vi "SM-SG Main.vi"() -> ()   [LabVIEW 2017]
doc: "Use this template to build a simple state machine design pattern. Each state executes code and determines which state to transition to."
uses:
  controls/SM-SG State.ctl
  controls/SM-SG Data.ctl
  <vilib>/Waveform/WDTOps.llb/WDT Append Waveforms DBL.vi
  <vilib>/measure/NI_MABase.lvlib
panel:
  in  "Parâmetros Onda Trapezoidal":T1
  in  "Parâmetros de Geração":T2
  in  "Configurações da Onda":T3
  out "Sinal":waveform(dbl)(graph)={"t0"=timestamp(0 s since 1904-01-01), "dt"=0.0002, "Y"=[]}
  out "Onda":dbl[](graph)
  in  "Abrir":bool
  in  "Salvar":bool
  in  "Limpa":bool
  in  "Adicionar":bool
  in  "Stop Button":bool
  # "Gerador de Sinais"
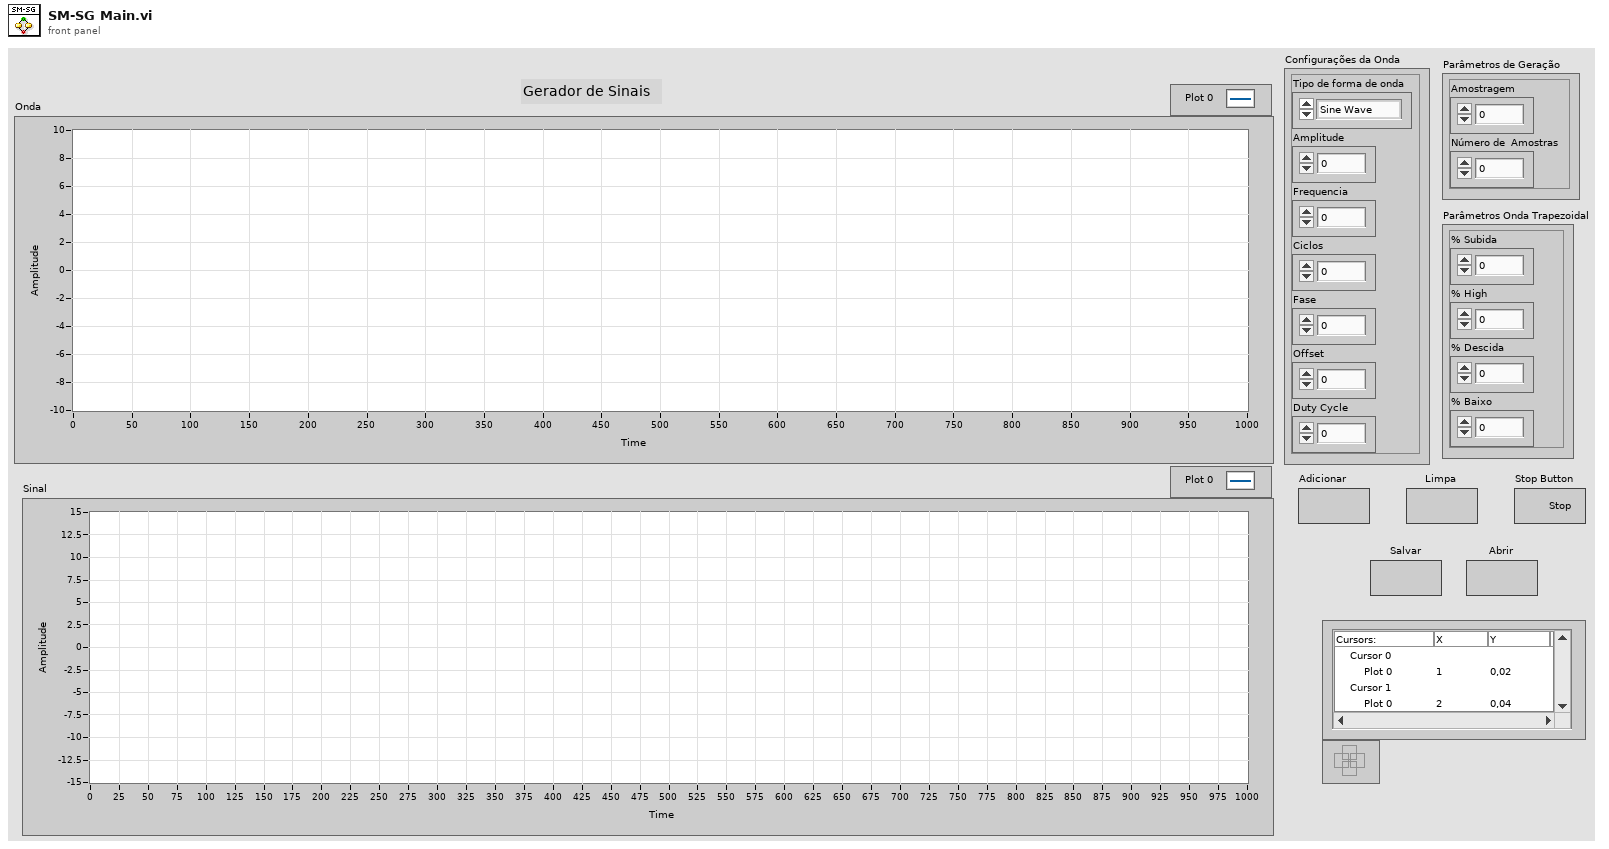
[diagram p1: front panel]
types:
  T1 = cluster{"% Subida ":dbl, "% High ":dbl, "% Descida ":dbl, "% Baixo":dbl}
  T2 = cluster{"Amostragem":dbl, "Número de  Amostras":dbl}
  T3 = cluster{"Tipo de forma de onda ":enum16{"Sine Wave", "Triangle Wave", "Square Wave", "Sawtooth Wave", "Trapezoidal Wave"}, "Amplitude ":dbl, "Frequencia ":dbl, "Ciclos ":dbl, "Fase ":dbl, "Offset":dbl, "Duty Cycle ":dbl}
  T4 = typedef "SM-SG Data.ctl" = cluster{"Onda":waveform(dbl), "Sinal":waveform(dbl), "Configurações\n da Onda":cluster{"Tipo de forma de onda ":enum16{"Sine Wave", "Triangle Wave", "Square Wave", "Sawtooth Wave", "Trapezoidal Wave"}, "Amplitude ":dbl, "Frequencia ":dbl, "Ciclos ":dbl, "Fase ":dbl, "Offset":dbl, "Duty Cycle ":dbl}, "Parâmetros de Geração":cluster{"Amostragem":dbl, "Número de  Amostras":dbl}, "Parâmetros Onda Trapezoidal":cluster{"% Subida ":dbl, "% High ":dbl, "% Descida ":dbl, "% Baixo":dbl}}
  T5 = typedef "SM-SG State.ctl" = enum16{"Inicio", "Aguarda Evento", "Desenha Onda", "Mostra Onda", "Mostra Sinal", "Limpa Gráfico", "Adicionar", "Remover", "Salvar", "Carregar", "Sair"}
  T6 = enum16{"Sine Wave", "Triangle Wave", "Square Wave", "Sawtooth Wave", "Trapezoidal Wave"}
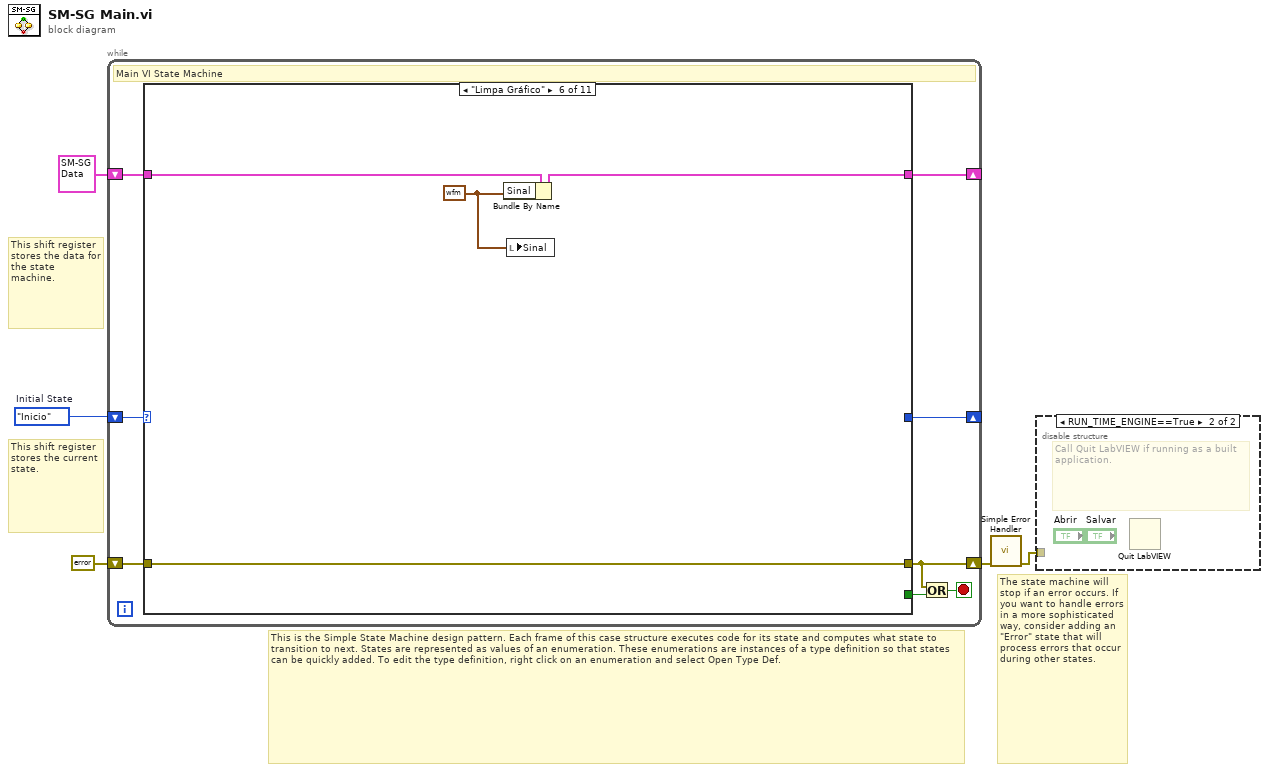
[diagram p0: block diagram]
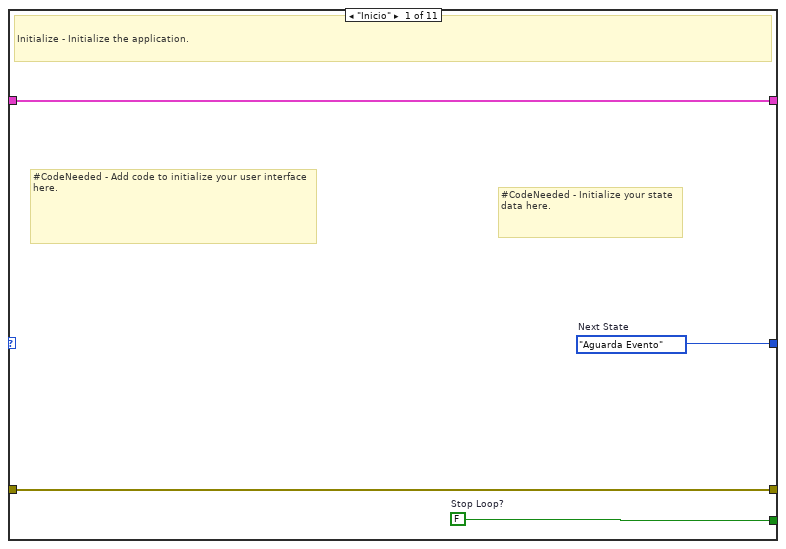
[diagram p3: hidden frame]
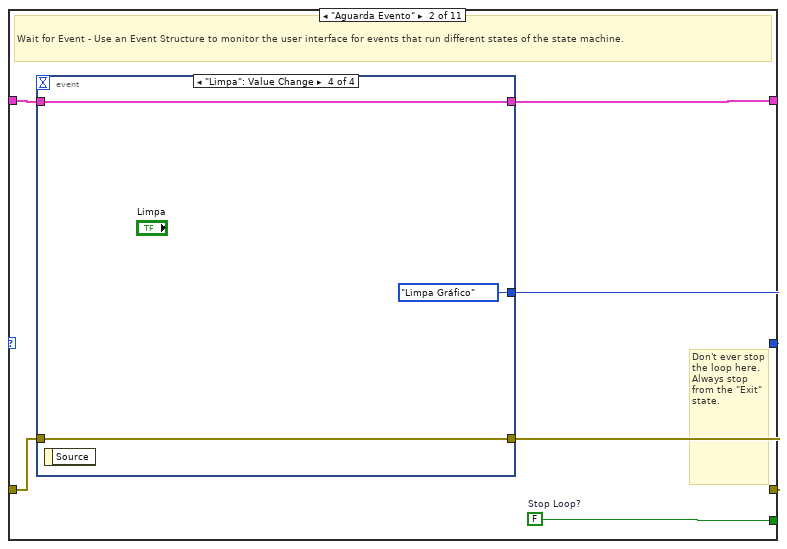
[diagram p4: hidden frame]
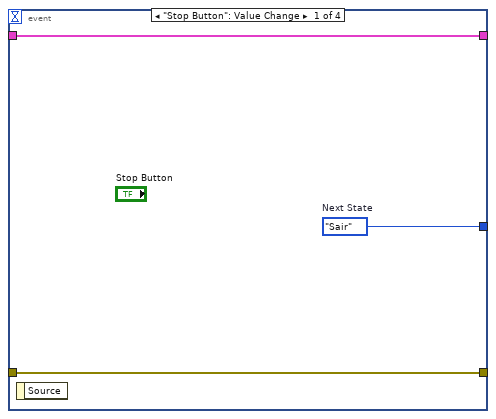
[diagram p5: hidden frame]
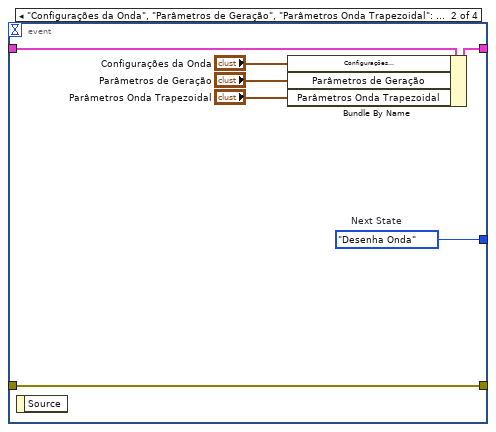
[diagram p6: hidden frame]
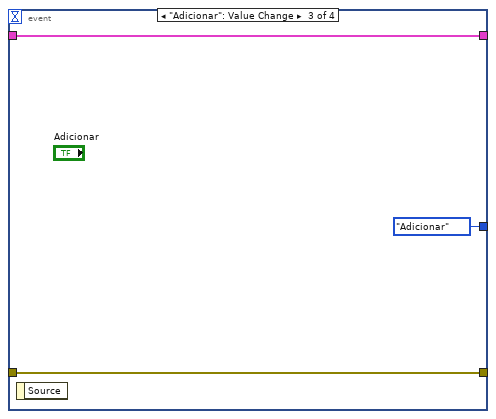
[diagram p7: hidden frame]
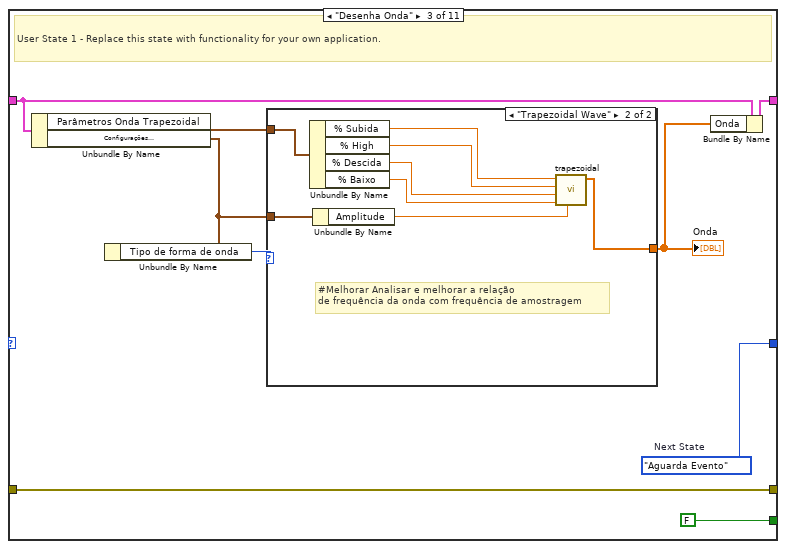
[diagram p8: hidden frame]
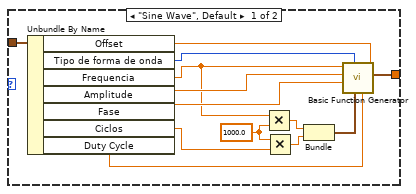
[diagram p9: hidden frame]
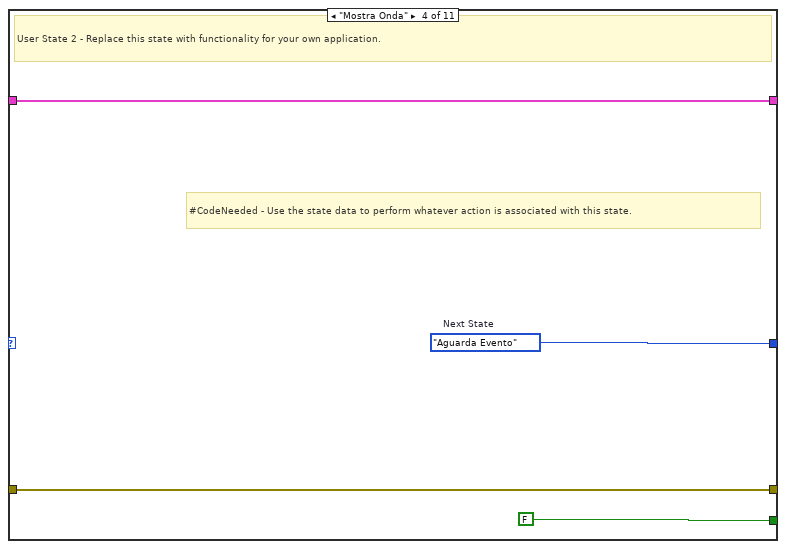
[diagram p10: hidden frame]
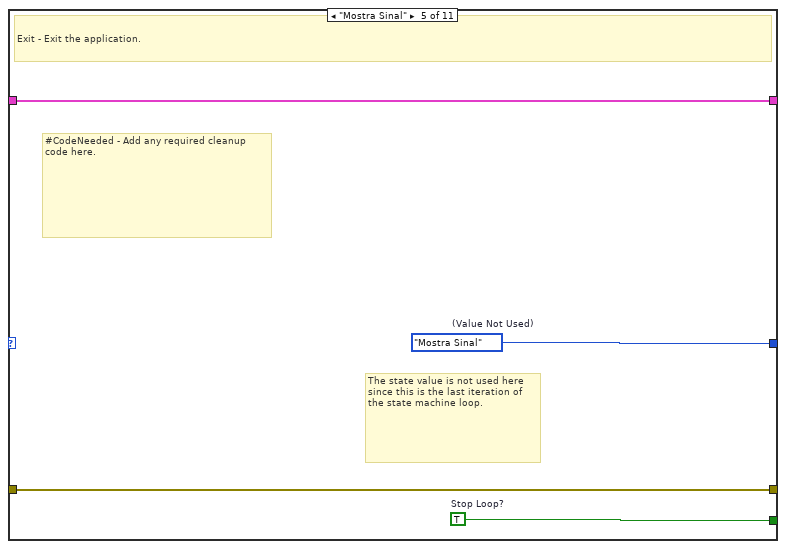
[diagram p11: hidden frame]
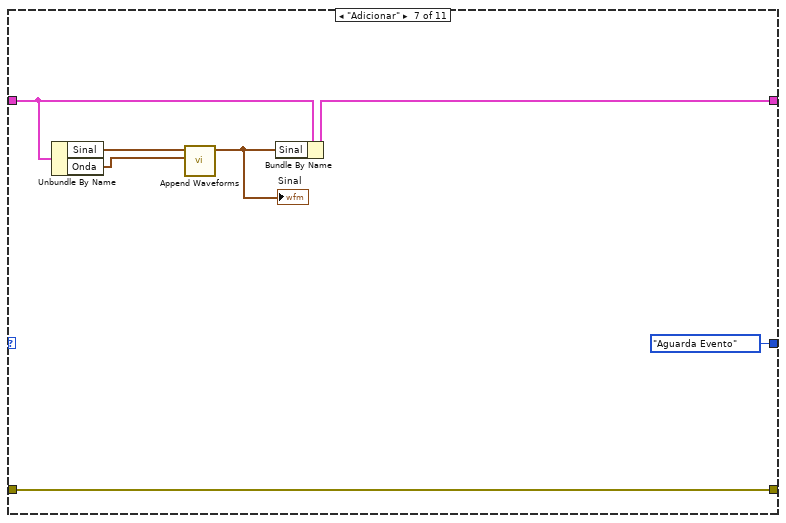
[diagram p12: hidden frame]
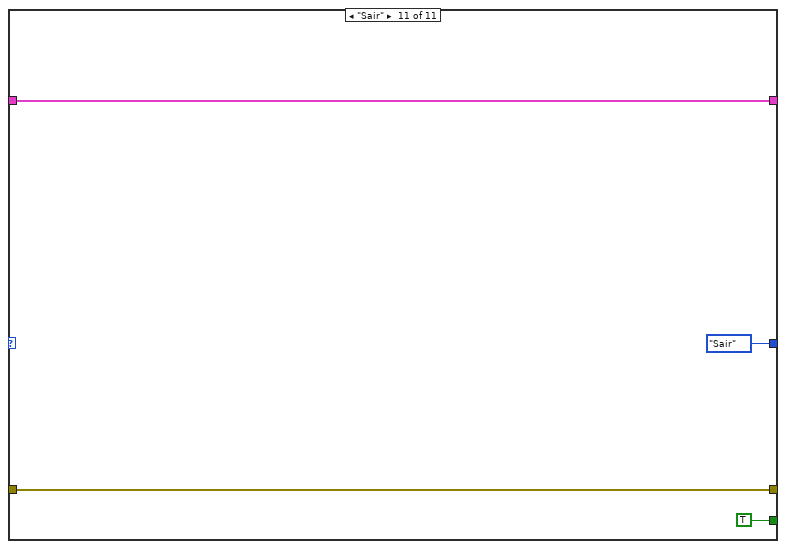
[diagram p16: hidden frame]
diagram:
  w5 = SM-SG_State."Inicio"  # Initial State
  # "The state machine will stop if an error occurs. If you want to handle errors in a more sophisticated way, consider adding an \"Error\" state that will process errors that occur during other states."
  # "This shift register stores the data for the state machine."
  # "This is the Simple State Machine design pattern. Each frame of this case structure executes code for its state and computes what state to transition to next. States are represented as values of an enumeration. These enumerations are instances of a type definition so that states can be quickly added. To edit the type definition, right click on an enumeration and select Open Type Def."
  # "This shift register stores the current state."
  n1 = while {
    shift-right: [w12] -> _
    shift-left: w5 -> [w13]
    shift-right: [w10] -> _
    shift-left: T4 {"Onda"={"t0"=timestamp(0 s since 1904-01-01), "dt"=1.0, "Y"=[]}, "Sinal"={"t0"=timestamp(0 s since 1904-01-01), "dt"=1.0, "Y"=[]}, "Configurações\n da Onda"={"Tipo de forma de onda "=enum."Sine Wave", "Amplitude "=0.0, "Frequencia "=0.0, "Ciclos "=1.0, "Fase "=0.0, "Offset"=0.0, "Duty Cycle "=0.0}, "Parâmetros de Geração"={"Amostragem"=0.0, "Número de  Amostras"=0.0}, "Parâmetros Onda Trapezoidal"={"% Subida "=0.0, "% High "=0.0, "% Descida "=0.0, "% Baixo"=0.0}} ("Data") -> [w11]
    shift-right: [w6] -> w2
    shift-left: errorcluster {"status"=FALSE, "code"=0, "source"=""} ("error constant") -> [w9]
    stop <- w7 stop-if-true
    # "Main VI State Machine"
    n2 = case shown="\"Limpa Gráfico\"" w13 {
      tunnel: [w17 w23 w48 w73 w77 _ SM-SG_State."Aguarda Evento" ("(Value Not Used)") _ _ _ SM-SG_State."Sair" ("(Value Not Used)")] -> w12
      tunnel: [w16 w22 FALSE ("Stop Loop?") FALSE ("Stop Loop?") w75 _ _ _ _ _ TRUE ("Stop Loop?")] -> w8
      tunnel: w11 -> [w15 w21 w43 w71 w76 w81 w87 w90 w92 w94 w98]
      tunnel: [w15 w20 w40 w71 w76 w79 w84 w90 w92 w94 w98] -> w10
      tunnel: w9 -> [w14 w19 w46 w70 w74 w80 w88 w89 w91 w93 w97]
      tunnel: [w14 w18 w46 w70 w74 w80 w88 w89 w91 w93 w97] -> w6
      frame "Inicio" {
        w16 = FALSE  # Stop Loop?
        w17 = SM-SG_State."Aguarda Evento"  # Next State
        # "#CodeNeeded - Initialize your state data here."
        # "#CodeNeeded - Add code to initialize your user interface here."
        # "Initialize - Initialize the application."
      }
      frame "Aguarda Evento" {
        w22 = FALSE  # Stop Loop?
        # "Don't ever stop the loop here. Always stop from the \"Exit\" state."
        # "Wait for Event - Use an Event Structure to monitor the user interface for events that run different states of the state machine."
        n3 = event shown="[3] \"Limpa\": Value Change" {
          selector: _ -> [_ _ _ _]
          dyn-events: _ -> [_ _ _ _]
          timeout: _ -> [_ _ _ _]
          tunnel: [w26 w33 SM-SG_State."Adicionar" ("Next State") SM-SG_State."Limpa Gráfico" ("Next State")] -> w23
          tunnel: w21 -> [w25 w32 w36 w39]
          tunnel: [w25 w31 w36 w39] -> w20
          tunnel: w19 -> [w24 w30 w35 w38]
          tunnel: [w24 w30 w35 w38] -> w18
          event "Stop Button": Value Change {
            w26 = SM-SG_State."Sair"  # Next State
            n4 = event-data() -> ()  [unwired: 1 in, 1 out]
          }
          event "Configurações da Onda", "Parâmetros de Geração", "Parâmetros Onda Trapezoidal": Value Change {
            w33 = SM-SG_State."Desenha Onda"  # Next State
            n5 = event-data() -> ()  [unwired: 1 in, 1 out]
            n6 = Bundle By Name(cluster=w32, "Configurações\n da Onda"="Configurações da Onda", "Parâmetros de Geração"="Parâmetros de Geração", "Parâmetros Onda Trapezoidal"="Parâmetros Onda Trapezoidal") -> (w31:T4)
          }
          event "Adicionar": Value Change {
            n7 = event-data() -> ()  [unwired: 1 in, 1 out]
          }
          event "Limpa": Value Change {
            n8 = event-data() -> ()  [unwired: 1 in, 1 out]
          }
        }
      }
      frame "Desenha Onda" {
        w48 = SM-SG_State."Aguarda Evento"  # Next State
        # "User State 1 - Replace this state with functionality for your own application."
        n9 = Unbundle By Name(w43) -> ("Parâmetros Onda Trapezoidal"=w42:T1, "Configurações\n da Onda"=w44:T3)
        n10 = Unbundle By Name(w44) -> ("Tipo de forma de onda"=w45:T6)
        n11 = case shown="\"Trapezoidal Wave\"" w45 {
          tunnel: w44 -> [w61 w69]
          tunnel: [w49 w62] -> w41
          tunnel: w42 -> [_ w68]
          frame "Sine Wave", Default {
            w53 = 1000.0 ("y")
            n12 = Unbundle By Name(w61) -> ("Offset"=w60:dbl, "Tipo de forma de onda"=w59:T6, "Frequencia"=w51:dbl, "Amplitude"=w58:dbl, "Fase"=w57:dbl, "Ciclos"=w52:dbl, "Duty Cycle"=w56:dbl)
            n13 = Multiply(x=w51, y=w53) -> (x*y=w54:dbl)
            n14 = Multiply(x=w53, y=w52) -> (x*y=w55:dbl)
            n15 = Bundle(w54, w55) -> (w50:cluster{dbl, dbl})  [unwired: 1 in]
            n16 = call <vilib>:"Basic Function Generator.vi"("offset"=w60, "square wave duty cycle (%)"=w56, "sampling info"=w50, "signal type"=w59, "phase"=w57, "amplitude"=w58, "frequency"=w51) -> ("signal out"=w49:waveform(dbl))  [unwired: 2 in, 2 out]
          }
          frame "Trapezoidal Wave" {
            # "#Melhorar Analisar e melhorar a relação\nde frequência da onda com frequência de amostragem"
            n17 = Unbundle By Name(w68) -> ("% Subida"=w67:dbl, "% High"=w66:dbl, "% Descida"=w65:dbl, "% Baixo"=w64:dbl)
            n18 = Unbundle By Name(w69) -> ("Amplitude"=w63:dbl)
            n19 = call "trapezoidal.vi"("Amplitude"=w63, "%Baixo"=w64, "%Descida"=w65, "%Alto"=w66, "%Subida"=w67) -> ("Waveform Graph"=w62:dbl[])  [unwired: 6 in]
          }
        }
        "Onda" <- w41
        n20 = Bundle By Name(cluster=w43, "Onda"=w41) -> (w40:T4)
      }
      frame "Mostra Onda" {
        w73 = SM-SG_State."Aguarda Evento"  # Next State
        # "#CodeNeeded - Use the state data to perform whatever action is associated with this state."
        # "User State 2 - Replace this state with functionality for your own application."
      }
      frame "Mostra Sinal" {
        w75 = TRUE  # Stop Loop?
        w77 = SM-SG_State."Mostra Sinal"  # (Value Not Used)
        # "#CodeNeeded - Add any required cleanup code here."
        # "The state value is not used here since this is the last iteration of the state machine loop."
        # "Exit - Exit the application."
      }
      frame "Limpa Gráfico" {
        w78 = waveform(dbl) {"t0"=timestamp(0 s since 1904-01-01), "dt"=1.0, "Y"=[]} ("Waveform")
        n21 = Bundle By Name(cluster=w81, "Sinal"=w78) -> (w79:T4)
        n22 = local write "Sinal"(w78) -> ()
      }
      frame "Adicionar" {
        n23 = Unbundle By Name(w87) -> ("Sinal"=w86:waveform(dbl), "Onda"=w85:waveform(dbl))
        n24 = call-poly <vilib>:"Append Waveforms.vi"("waveform B"=w85, "waveform A"=w86) -> ("waveform out"=w83:waveform(dbl))  [unwired: 8 in, 1 out]
        "Sinal" <- w83
        n25 = Bundle By Name(cluster=w87, "Sinal"=w83) -> (w84:T4)
      }
      frame "Remover" {
      }
      frame "Salvar" {
      }
      frame "Carregar" {
      }
      frame "Sair" {
      }
    }
    n26 = Or(x=w6, y=w8) -> (x .or. y?=w7:bool)
  }
  n27 = call <vilib>:"Simple Error Handler.vi"("error in (no error)"=w2) -> ("error out"=w1:errorcluster)  [unwired: 4 in, 4 out]
  n28 = disable-structure shown="RUN_TIME_ENGINE==True" {
    disable-tunnel: w1 -> [_ _]
    frame condition #0 (active) {
    }
    frame condition #1 {
      # "Call Quit LabVIEW if running as a built application."
      n29 = Quit LabVIEW() -> ()  [unwired: 1 in]
    }
  }
